vi "Send Configure Edge Trigger Source.vi"(6 "trigger level  (0.0 V)":dbl[unit] format="%.3f", 7 "Message Priority (Normal)":T1=enum."Normal", 8 "error in (no error)":errorcluster, 9 "trigger slope (Positive)":i32(ring)=1 items=["Positive"=1, "Negative"=0], 10 "trigger source (CHANNEL1)":string(combo)="CHANNEL1" caption="trigger source (\"CHANNEL1\")", 11 "Message Enqueuer":refnum<class "Message Enqueuer.lvclass">) -> (0 "error out":errorcluster, 3 "Message Enqueuer out":refnum<class "Message Enqueuer.lvclass">)   [LabVIEW 2015, in "CS++Scope.lvlib" / "Configure Edge Trigger Source Msg.lvclass"]
doc: "Sends the <B>CS++Scope.lvlib:Configure Edge Trigger Source Msg.lvclass</B> message.\n\n<B>CS++Scope.lvlib:CS++Scope.lvclass:Configure Edge Trigger Source.vi</B> Description:\n\nThis VI configures the edge trigger. An edge trigger occurs when the trigger signal passes through the voltage threshold that you specify with the Trigger Level parameter and has the slope that you specify with the Trigger Slope parameter. \n\nNotes:\n (1) This VI affects instrument behavior only if the trigger type is\n IVISCOPE_VAL_EDGE_TRIGGER. Call the IviScope Configure Trigger and\n IviScope Configure Trigger Coupling VIs to set the trigger type and trigger coupling\n before calling this VI.\n (2) If the trigger source is one of the analog input channels, you must configure\n the vertical range, vertical offset, vertical coupling, probe attenuation, and the\n maximum input frequency before calling this VI."
uses:
  Configure Edge Trigger Source Msg.lvclass
  <vilib>/ActorFramework/Message Enqueuer/Message Enqueuer.lvclass
  <vilib>/ActorFramework/Message Enqueuer/Message Priority.ctl
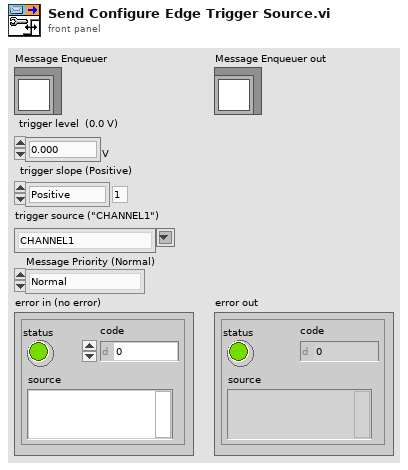
[diagram p1: front panel]
types:
  T1 = typedef "Actor Framework.lvlib/Message Enqueuer.lvclass/Message Priority.ctl" = enum16{"Low", "Normal", "High"}
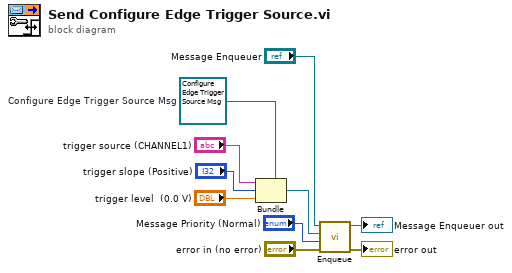
[diagram p0: block diagram]
diagram:
  w4 = refnum<class "Configure Edge Trigger Source Msg.lvclass"> refnum  # Configure Edge Trigger Source Msg
  n1 = Bundle(cluster=w4, "trigger source (CHANNEL1)", "trigger slope (Positive)", "trigger level  (0.0 V)") -> (w7:refnum<class "Configure Edge Trigger Source Msg.lvclass">)
  n2 = call <vilib>:"Enqueue.vi"("error in (no error)"="error in (no error)", "Message Priority (Normal)"="Message Priority (Normal)", "Message"=w7, "Message Enqueuer in"="Message Enqueuer") -> ("error out"=→"error out":errorcluster, "Message Enqueuer out"=→"Message Enqueuer out":refnum<class "Message Enqueuer.lvclass">)  [unwired: 6 in]
